vi "ReadData_9234.vi"(8 "error in":errorcluster, 11 "Module Config Selector":i16) -> (0 "error out":errorcluster, 3 "Data Array":sgl[](array[numeric]) format="%.2f")   [LabVIEW 2017, in "BOP_VibAPI_8.lvlib"]
uses:
  <vilib>/addons/InsightCM/Devices/Shared/Cms/Fpga/Acquisition/source/subVIs/VibAPI_8/BOP_VibAPI_8.lvlib
  <vilib>/rvi/eio/common/nirviEmuTemplateMethod_errors.vi
  <vilib>/eio/EIONode/EIONode.xnode
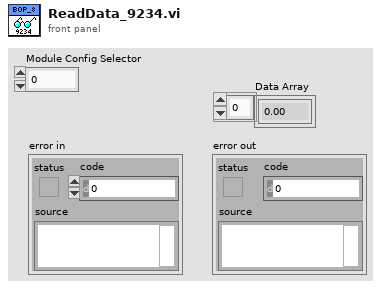
[diagram p1: front panel]
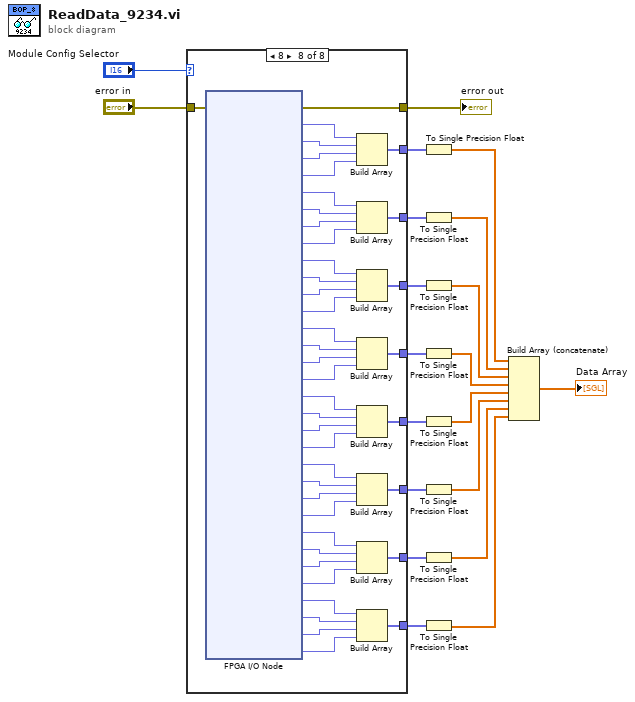
[diagram p0: block diagram]
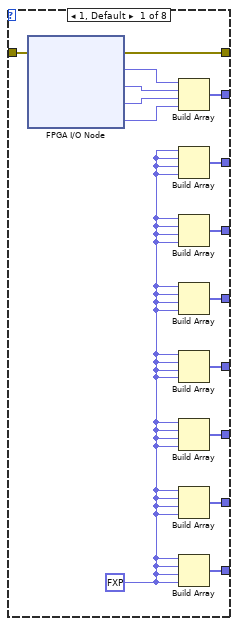
[diagram p2: hidden frame]
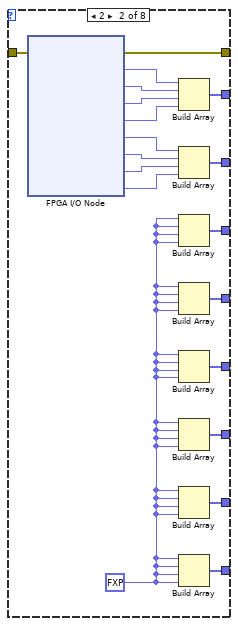
[diagram p3: hidden frame]
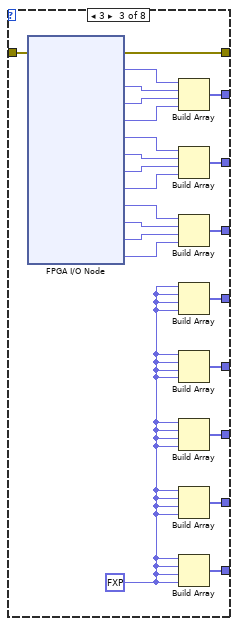
[diagram p4: hidden frame]
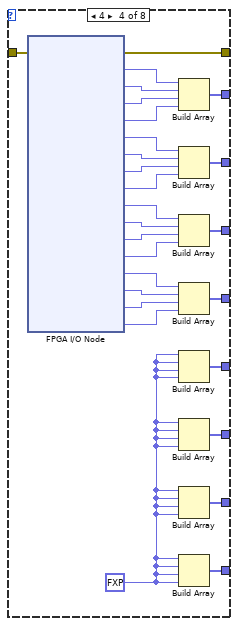
[diagram p5: hidden frame]
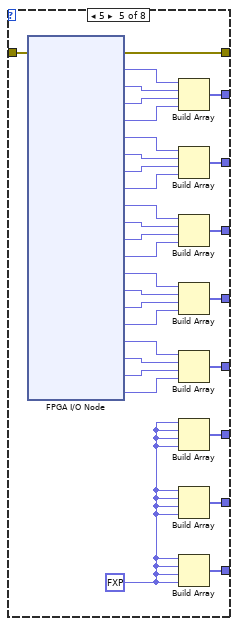
[diagram p6: hidden frame]
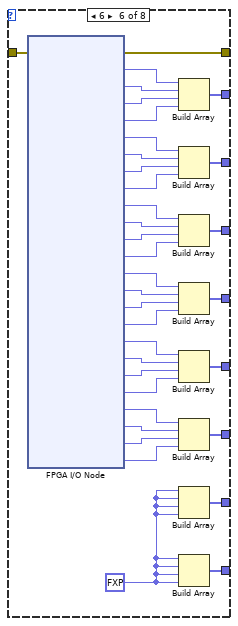
[diagram p7: hidden frame]
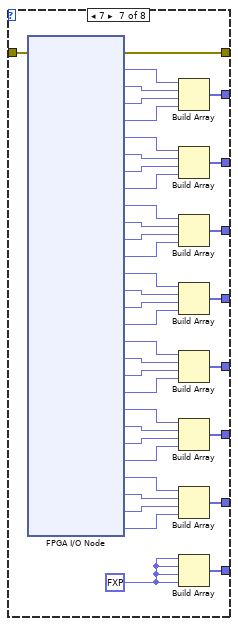
[diagram p8: hidden frame]
diagram:
  n1 = case shown="8" "Module Config Selector" {
    tunnel: "error in" -> [w32 w51 w74 w101 w132 w167 w206 w248]
    tunnel: [w31 w50 w73 w100 w131 w166 w205 w247] -> w5
    tunnel: [w30 w49 w72 w99 w130 w165 w204 w246] -> w9
    tunnel: [w29 w48 w71 w98 w129 w164 w203 w245] -> w11
    tunnel: [w28 w47 w70 w97 w128 w163 w202 w244] -> w12
    tunnel: [w24 w39 w58 w96 w127 w162 w201 w243] -> w13
    tunnel: [w27 w46 w69 w95 w126 w161 w200 w242] -> w14
    tunnel: [w26 w45 w68 w94 w125 w160 w199 w241] -> w15
    tunnel: [w23 w37 w56 w79 w106 w137 w177 w219] -> w4
    tunnel: [w22 w36 w55 w78 w105 w136 w171 w214] -> w3
    frame 1, Default {
      w21 = fxp<+/-,24,7> 0.0 ("Mod1/AI2")
      n2 = xnode "FPGA I/O Node"("error in"=w32) -> ("error out"=w31:errorcluster, "Mod1/AI0"=w33:fxp<+/-,24,4>, "Mod1/AI1"=w35:fxp<+/-,24,4>, "Mod1/AI2"=w34:fxp<+/-,24,4>, "Mod1/AI3"=w25:fxp<+/-,24,4>)  [unwired: 4 in, 4 out]
      n3 = Build Array(w33, w35, w34, w25) -> (w30:fxp<+/-,24,4>[])
      n4 = Build Array(w21, w21, w21, w21) -> (w29:fxp<+/-,24,7>[])
      n5 = Build Array(w21, w21, w21, w21) -> (w28:fxp<+/-,24,7>[])
      n6 = Build Array(w21, w21, w21, w21) -> (w24:fxp<+/-,24,7>[])
      n7 = Build Array(w21, w21, w21, w21) -> (w27:fxp<+/-,24,7>[])
      n8 = Build Array(w21, w21, w21, w21) -> (w26:fxp<+/-,24,7>[])
      n9 = Build Array(w21, w21, w21, w21) -> (w23:fxp<+/-,24,7>[])
      n10 = Build Array(w21, w21, w21, w21) -> (w22:fxp<+/-,24,7>[])
    }
    frame 2 {
      w38 = fxp<+/-,24,7> 0.0 ("Mod1/AI2")
      n11 = xnode "FPGA I/O Node"("error in"=w51) -> ("error out"=w50:errorcluster, "Mod1/AI0"=w52:fxp<+/-,24,4>, "Mod1/AI1"=w54:fxp<+/-,24,4>, "Mod1/AI2"=w53:fxp<+/-,24,4>, "Mod1/AI3"=w41:fxp<+/-,24,4>, "Mod2/AI0"=w44:fxp<+/-,24,4>, "Mod2/AI1"=w43:fxp<+/-,24,4>, "Mod2/AI2"=w42:fxp<+/-,24,4>, "Mod2/AI3"=w40:fxp<+/-,24,4>)  [unwired: 8 in, 8 out]
      n12 = Build Array(w52, w54, w53, w41) -> (w49:fxp<+/-,24,4>[])
      n13 = Build Array(w44, w43, w42, w40) -> (w48:fxp<+/-,24,4>[])
      n14 = Build Array(w38, w38, w38, w38) -> (w47:fxp<+/-,24,7>[])
      n15 = Build Array(w38, w38, w38, w38) -> (w39:fxp<+/-,24,7>[])
      n16 = Build Array(w38, w38, w38, w38) -> (w46:fxp<+/-,24,7>[])
      n17 = Build Array(w38, w38, w38, w38) -> (w45:fxp<+/-,24,7>[])
      n18 = Build Array(w38, w38, w38, w38) -> (w37:fxp<+/-,24,7>[])
      n19 = Build Array(w38, w38, w38, w38) -> (w36:fxp<+/-,24,7>[])
    }
    frame 3 {
      w57 = fxp<+/-,24,7> 0.0 ("Mod1/AI2")
      n20 = xnode "FPGA I/O Node"("error in"=w74) -> ("error out"=w73:errorcluster, "Mod1/AI0"=w75:fxp<+/-,24,4>, "Mod1/AI1"=w77:fxp<+/-,24,4>, "Mod1/AI2"=w76:fxp<+/-,24,4>, "Mod1/AI3"=w61:fxp<+/-,24,4>, "Mod2/AI0"=w67:fxp<+/-,24,4>, "Mod2/AI1"=w66:fxp<+/-,24,4>, "Mod2/AI2"=w65:fxp<+/-,24,4>, "Mod2/AI3"=w59:fxp<+/-,24,4>, "Mod3/AI0"=w64:fxp<+/-,24,4>, "Mod3/AI1"=w63:fxp<+/-,24,4>, "Mod3/AI2"=w62:fxp<+/-,24,4>, "Mod3/AI3"=w60:fxp<+/-,24,4>)  [unwired: 12 in, 12 out]
      n21 = Build Array(w75, w77, w76, w61) -> (w72:fxp<+/-,24,4>[])
      n22 = Build Array(w67, w66, w65, w59) -> (w71:fxp<+/-,24,4>[])
      n23 = Build Array(w64, w63, w62, w60) -> (w70:fxp<+/-,24,4>[])
      n24 = Build Array(w57, w57, w57, w57) -> (w58:fxp<+/-,24,7>[])
      n25 = Build Array(w57, w57, w57, w57) -> (w69:fxp<+/-,24,7>[])
      n26 = Build Array(w57, w57, w57, w57) -> (w68:fxp<+/-,24,7>[])
      n27 = Build Array(w57, w57, w57, w57) -> (w56:fxp<+/-,24,7>[])
      n28 = Build Array(w57, w57, w57, w57) -> (w55:fxp<+/-,24,7>[])
    }
    frame 4 {
      w80 = fxp<+/-,24,7> 0.0 ("Mod1/AI2")
      n29 = xnode "FPGA I/O Node"("error in"=w101) -> ("error out"=w100:errorcluster, "Mod1/AI0"=w102:fxp<+/-,24,4>, "Mod1/AI1"=w104:fxp<+/-,24,4>, "Mod1/AI2"=w103:fxp<+/-,24,4>, "Mod1/AI3"=w84:fxp<+/-,24,4>, "Mod2/AI0"=w93:fxp<+/-,24,4>, "Mod2/AI1"=w92:fxp<+/-,24,4>, "Mod2/AI2"=w91:fxp<+/-,24,4>, "Mod2/AI3"=w81:fxp<+/-,24,4>, "Mod3/AI0"=w90:fxp<+/-,24,4>, "Mod3/AI1"=w89:fxp<+/-,24,4>, "Mod3/AI2"=w88:fxp<+/-,24,4>, "Mod3/AI3"=w82:fxp<+/-,24,4>, "Mod4/AI0"=w87:fxp<+/-,24,4>, "Mod4/AI1"=w86:fxp<+/-,24,4>, "Mod4/AI2"=w85:fxp<+/-,24,4>, "Mod4/AI3"=w83:fxp<+/-,24,4>)  [unwired: 16 in, 16 out]
      n30 = Build Array(w102, w104, w103, w84) -> (w99:fxp<+/-,24,4>[])
      n31 = Build Array(w93, w92, w91, w81) -> (w98:fxp<+/-,24,4>[])
      n32 = Build Array(w90, w89, w88, w82) -> (w97:fxp<+/-,24,4>[])
      n33 = Build Array(w87, w86, w85, w83) -> (w96:fxp<+/-,24,4>[])
      n34 = Build Array(w80, w80, w80, w80) -> (w95:fxp<+/-,24,7>[])
      n35 = Build Array(w80, w80, w80, w80) -> (w94:fxp<+/-,24,7>[])
      n36 = Build Array(w80, w80, w80, w80) -> (w79:fxp<+/-,24,7>[])
      n37 = Build Array(w80, w80, w80, w80) -> (w78:fxp<+/-,24,7>[])
    }
    frame 5 {
      w107 = fxp<+/-,24,7> 0.0 ("Mod1/AI2")
      n38 = xnode "FPGA I/O Node"("error in"=w132) -> ("error out"=w131:errorcluster, "Mod1/AI0"=w133:fxp<+/-,24,4>, "Mod1/AI1"=w135:fxp<+/-,24,4>, "Mod1/AI2"=w134:fxp<+/-,24,4>, "Mod1/AI3"=w112:fxp<+/-,24,4>, "Mod2/AI0"=w124:fxp<+/-,24,4>, "Mod2/AI1"=w123:fxp<+/-,24,4>, "Mod2/AI2"=w122:fxp<+/-,24,4>, "Mod2/AI3"=w108:fxp<+/-,24,4>, "Mod3/AI0"=w121:fxp<+/-,24,4>, "Mod3/AI1"=w120:fxp<+/-,24,4>, "Mod3/AI2"=w119:fxp<+/-,24,4>, "Mod3/AI3"=w109:fxp<+/-,24,4>, "Mod4/AI0"=w118:fxp<+/-,24,4>, "Mod4/AI1"=w117:fxp<+/-,24,4>, "Mod4/AI2"=w116:fxp<+/-,24,4>, "Mod4/AI3"=w110:fxp<+/-,24,4>, "Mod5/AI0"=w115:fxp<+/-,24,4>, "Mod5/AI1"=w114:fxp<+/-,24,4>, "Mod5/AI2"=w113:fxp<+/-,24,4>, "Mod5/AI3"=w111:fxp<+/-,24,4>)  [unwired: 20 in, 20 out]
      n39 = Build Array(w133, w135, w134, w112) -> (w130:fxp<+/-,24,4>[])
      n40 = Build Array(w124, w123, w122, w108) -> (w129:fxp<+/-,24,4>[])
      n41 = Build Array(w121, w120, w119, w109) -> (w128:fxp<+/-,24,4>[])
      n42 = Build Array(w118, w117, w116, w110) -> (w127:fxp<+/-,24,4>[])
      n43 = Build Array(w115, w114, w113, w111) -> (w126:fxp<+/-,24,4>[])
      n44 = Build Array(w107, w107, w107, w107) -> (w125:fxp<+/-,24,7>[])
      n45 = Build Array(w107, w107, w107, w107) -> (w106:fxp<+/-,24,7>[])
      n46 = Build Array(w107, w107, w107, w107) -> (w105:fxp<+/-,24,7>[])
    }
    frame 6 {
      w138 = fxp<+/-,24,7> 0.0 ("Mod1/AI2")
      n47 = xnode "FPGA I/O Node"("error in"=w167) -> ("error out"=w166:errorcluster, "Mod1/AI0"=w168:fxp<+/-,24,4>, "Mod1/AI1"=w170:fxp<+/-,24,4>, "Mod1/AI2"=w169:fxp<+/-,24,4>, "Mod1/AI3"=w144:fxp<+/-,24,4>, "Mod2/AI0"=w159:fxp<+/-,24,4>, "Mod2/AI1"=w158:fxp<+/-,24,4>, "Mod2/AI2"=w157:fxp<+/-,24,4>, "Mod2/AI3"=w139:fxp<+/-,24,4>, "Mod3/AI0"=w156:fxp<+/-,24,4>, "Mod3/AI1"=w155:fxp<+/-,24,4>, "Mod3/AI2"=w154:fxp<+/-,24,4>, "Mod3/AI3"=w140:fxp<+/-,24,4>, "Mod4/AI0"=w153:fxp<+/-,24,4>, "Mod4/AI1"=w152:fxp<+/-,24,4>, "Mod4/AI2"=w151:fxp<+/-,24,4>, "Mod4/AI3"=w141:fxp<+/-,24,4>, "Mod5/AI0"=w150:fxp<+/-,24,4>, "Mod5/AI1"=w149:fxp<+/-,24,4>, "Mod5/AI2"=w148:fxp<+/-,24,4>, "Mod5/AI3"=w142:fxp<+/-,24,4>, "Mod6/AI0"=w147:fxp<+/-,24,4>, "Mod6/AI1"=w146:fxp<+/-,24,4>, "Mod6/AI2"=w145:fxp<+/-,24,4>, "Mod6/AI3"=w143:fxp<+/-,24,4>)  [unwired: 24 in, 24 out]
      n48 = Build Array(w168, w170, w169, w144) -> (w165:fxp<+/-,24,4>[])
      n49 = Build Array(w159, w158, w157, w139) -> (w164:fxp<+/-,24,4>[])
      n50 = Build Array(w156, w155, w154, w140) -> (w163:fxp<+/-,24,4>[])
      n51 = Build Array(w153, w152, w151, w141) -> (w162:fxp<+/-,24,4>[])
      n52 = Build Array(w150, w149, w148, w142) -> (w161:fxp<+/-,24,4>[])
      n53 = Build Array(w147, w146, w145, w143) -> (w160:fxp<+/-,24,4>[])
      n54 = Build Array(w138, w138, w138, w138) -> (w137:fxp<+/-,24,7>[])
      n55 = Build Array(w138, w138, w138, w138) -> (w136:fxp<+/-,24,7>[])
    }
    frame 7 {
      w172 = fxp<+/-,24,7> 0.0 ("Mod1/AI2")
      n56 = xnode "FPGA I/O Node"("error in"=w206) -> ("error out"=w205:errorcluster, "Mod1/AI0"=w207:fxp<+/-,24,4>, "Mod1/AI1"=w209:fxp<+/-,24,4>, "Mod1/AI2"=w208:fxp<+/-,24,4>, "Mod1/AI3"=w183:fxp<+/-,24,4>, "Mod2/AI0"=w198:fxp<+/-,24,4>, "Mod2/AI1"=w197:fxp<+/-,24,4>, "Mod2/AI2"=w196:fxp<+/-,24,4>, "Mod2/AI3"=w178:fxp<+/-,24,4>, "Mod3/AI0"=w195:fxp<+/-,24,4>, "Mod3/AI1"=w194:fxp<+/-,24,4>, "Mod3/AI2"=w193:fxp<+/-,24,4>, "Mod3/AI3"=w179:fxp<+/-,24,4>, "Mod4/AI0"=w192:fxp<+/-,24,4>, "Mod4/AI1"=w191:fxp<+/-,24,4>, "Mod4/AI2"=w190:fxp<+/-,24,4>, "Mod4/AI3"=w180:fxp<+/-,24,4>, "Mod5/AI0"=w189:fxp<+/-,24,4>, "Mod5/AI1"=w188:fxp<+/-,24,4>, "Mod5/AI2"=w187:fxp<+/-,24,4>, "Mod5/AI3"=w181:fxp<+/-,24,4>, "Mod6/AI0"=w186:fxp<+/-,24,4>, "Mod6/AI1"=w185:fxp<+/-,24,4>, "Mod6/AI2"=w184:fxp<+/-,24,4>, "Mod6/AI3"=w182:fxp<+/-,24,4>, "Mod7/AI0"=w176:fxp<+/-,24,4>, "Mod7/AI1"=w173:fxp<+/-,24,4>, "Mod7/AI2"=w174:fxp<+/-,24,4>, "Mod7/AI3"=w175:fxp<+/-,24,4>)  [unwired: 28 in, 28 out]
      n57 = Build Array(w207, w209, w208, w183) -> (w204:fxp<+/-,24,4>[])
      n58 = Build Array(w198, w197, w196, w178) -> (w203:fxp<+/-,24,4>[])
      n59 = Build Array(w195, w194, w193, w179) -> (w202:fxp<+/-,24,4>[])
      n60 = Build Array(w192, w191, w190, w180) -> (w201:fxp<+/-,24,4>[])
      n61 = Build Array(w189, w188, w187, w181) -> (w200:fxp<+/-,24,4>[])
      n62 = Build Array(w186, w185, w184, w182) -> (w199:fxp<+/-,24,4>[])
      n63 = Build Array(w176, w173, w174, w175) -> (w177:fxp<+/-,24,4>[])
      n64 = Build Array(w172, w172, w172, w172) -> (w171:fxp<+/-,24,7>[])
    }
    frame 8 {
      n65 = xnode "FPGA I/O Node"("error in"=w248) -> ("error out"=w247:errorcluster, "Mod1/AI0"=w249:fxp<+/-,24,4>, "Mod1/AI1"=w251:fxp<+/-,24,4>, "Mod1/AI2"=w250:fxp<+/-,24,4>, "Mod1/AI3"=w225:fxp<+/-,24,4>, "Mod2/AI0"=w240:fxp<+/-,24,4>, "Mod2/AI1"=w239:fxp<+/-,24,4>, "Mod2/AI2"=w238:fxp<+/-,24,4>, "Mod2/AI3"=w220:fxp<+/-,24,4>, "Mod3/AI0"=w237:fxp<+/-,24,4>, "Mod3/AI1"=w236:fxp<+/-,24,4>, "Mod3/AI2"=w235:fxp<+/-,24,4>, "Mod3/AI3"=w221:fxp<+/-,24,4>, "Mod4/AI0"=w234:fxp<+/-,24,4>, "Mod4/AI1"=w233:fxp<+/-,24,4>, "Mod4/AI2"=w232:fxp<+/-,24,4>, "Mod4/AI3"=w222:fxp<+/-,24,4>, "Mod5/AI0"=w231:fxp<+/-,24,4>, "Mod5/AI1"=w230:fxp<+/-,24,4>, "Mod5/AI2"=w229:fxp<+/-,24,4>, "Mod5/AI3"=w223:fxp<+/-,24,4>, "Mod6/AI0"=w228:fxp<+/-,24,4>, "Mod6/AI1"=w227:fxp<+/-,24,4>, "Mod6/AI2"=w226:fxp<+/-,24,4>, "Mod6/AI3"=w224:fxp<+/-,24,4>, "Mod7/AI0"=w218:fxp<+/-,24,4>, "Mod7/AI1"=w215:fxp<+/-,24,4>, "Mod7/AI2"=w216:fxp<+/-,24,4>, "Mod7/AI3"=w217:fxp<+/-,24,4>, "Mod8/AI0"=w212:fxp<+/-,24,4>, "Mod8/AI1"=w211:fxp<+/-,24,4>, "Mod8/AI2"=w210:fxp<+/-,24,4>, "Mod8/AI3"=w213:fxp<+/-,24,4>)  [unwired: 32 in, 32 out]
      n66 = Build Array(w249, w251, w250, w225) -> (w246:fxp<+/-,24,4>[])
      n67 = Build Array(w240, w239, w238, w220) -> (w245:fxp<+/-,24,4>[])
      n68 = Build Array(w237, w236, w235, w221) -> (w244:fxp<+/-,24,4>[])
      n69 = Build Array(w234, w233, w232, w222) -> (w243:fxp<+/-,24,4>[])
      n70 = Build Array(w231, w230, w229, w223) -> (w242:fxp<+/-,24,4>[])
      n71 = Build Array(w228, w227, w226, w224) -> (w241:fxp<+/-,24,4>[])
      n72 = Build Array(w218, w215, w216, w217) -> (w219:fxp<+/-,24,4>[])
      n73 = Build Array(w212, w211, w210, w213) -> (w214:fxp<+/-,24,4>[])
    }
  }
  "error out" <- w5
  n74 = To Single Precision Float(number=w9) -> (single precision float=w10:sgl[])
  n75 = To Single Precision Float(number=w11) -> (single precision float=w16:sgl[])
  n76 = To Single Precision Float(number=w12) -> (single precision float=w17:sgl[])
  n77 = To Single Precision Float(number=w13) -> (single precision float=w18:sgl[])
  n78 = To Single Precision Float(number=w14) -> (single precision float=w19:sgl[])
  n79 = To Single Precision Float(number=w15) -> (single precision float=w20:sgl[])
  n80 = To Single Precision Float(number=w4) -> (single precision float=w2:sgl[])
  n81 = To Single Precision Float(number=w3) -> (single precision float=w1:sgl[])
  n82 = Build Array (concatenate)(w10, w16, w17, w18, w19, w20, w2, w1) -> (→"Data Array":sgl[])
